vi "CRYIcon Setup.vi"(6 "error in (no error)":errorcluster, 9 "TS Tree In":refnum<vi>) -> (0 "error out":errorcluster, 3 "Tree ref":refnum<vi>)   [LabVIEW 2013]
doc: "This VI is designed to show how to use tree control methods and properties to perform the following high-level tasks:\n\n1. Use custom symbols for your tree control items.\n2. Traverse an already existing tree in a breadth-first fashion.\n\nRefer to the block diagram and subVI block diagram for implementation."
uses:
  CRYMainGlobal.vi
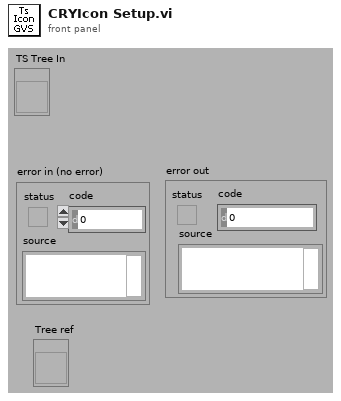
[diagram p1: front panel]
types:
  T1 = typedef "CRYImageData.ctl" = cluster{"image type":i32, "image depth":i32, "image":u8[], "mask":u8[], "colors":u32[], "Rectangle":cluster{"left":i16, "top":i16, "right":i16, "bottom":i16}}
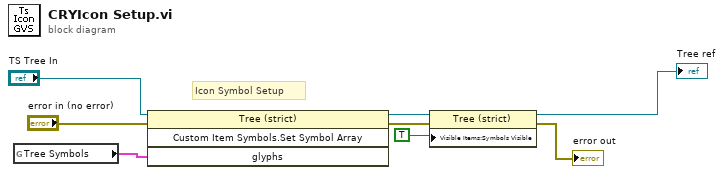
[diagram p0: block diagram]
diagram:
  # "Icon Symbol Setup"
  n1 = global read "CRYMainGlobal.vi" "Tree Symbols"() -> (w2:T1[])
  n2 = invoke class="Tree (strict)" method="Custom Item Symbols.Set Symbol Array"(reference="TS Tree In", error in="error in (no error)", "glyphs"=w2) -> (reference out=w6:refnum<vi>, error out=w3:errorcluster)  [unwired: 1 in, 2 out]
  n3 = property class="Tree (strict)"(reference=w6, error in=w3, "Visible Items:Symbols Visible"=TRUE) -> (reference out=→"Tree ref":refnum<vi>, error out=→"error out":errorcluster)
